vi "HEWH Close RLT Equipmet.vi"(7 "Semiphore":T1, 8 "Error In":errorcluster, 11 "RLT Equipment":T2={"COM A"="COM3", "MW100"="MW100", "AG34970"="A-34972A", "COM B"="COM4", "COM C"="COM5", "COM D"="COM6"}) -> (0 "Error Out":errorcluster)   [LabVIEW 2012]
uses:
  Drivers/Agilent 34970/Agilent 34970.lvlib
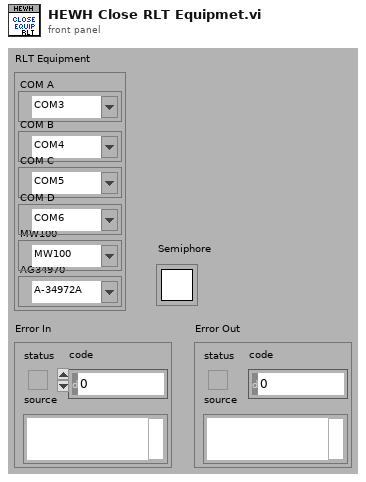
[diagram p1: front panel]
types:
  T1 = typedef "Semaphore RefNum" = refnum<k1>
  T2 = cluster{"COM A":refnum<visa-resource-name>, "MW100":refnum<visa-resource-name>, "AG34970":refnum<visa-resource-name>, "COM B":refnum<visa-resource-name>, "COM C":refnum<visa-resource-name>, "COM D":refnum<visa-resource-name>}
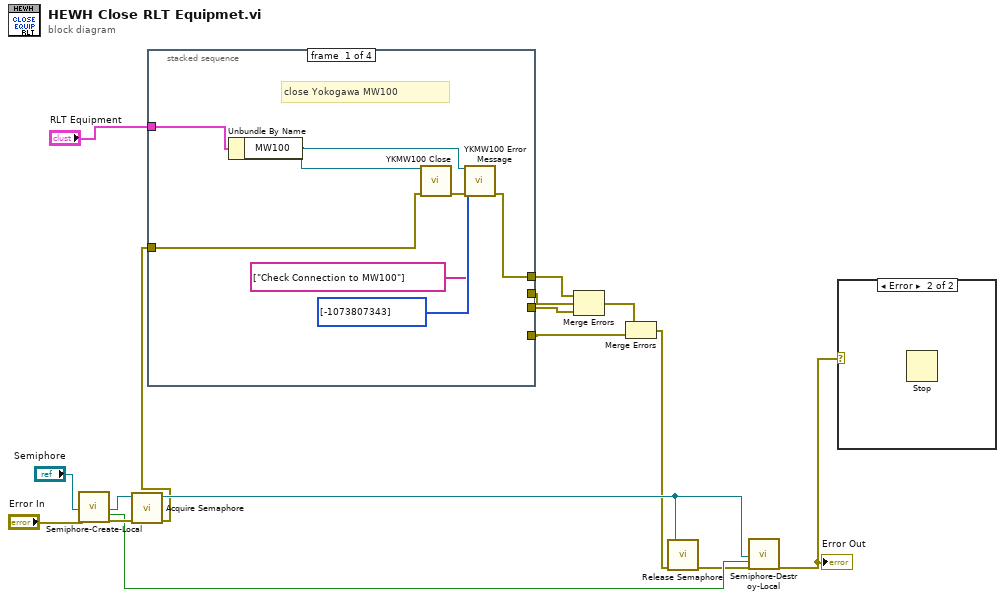
[diagram p0: block diagram]
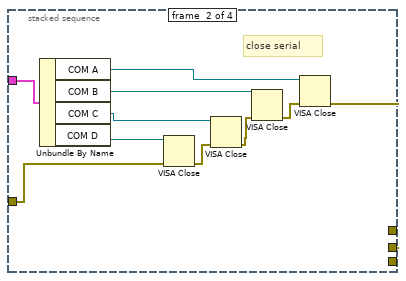
[diagram p3: hidden frame]
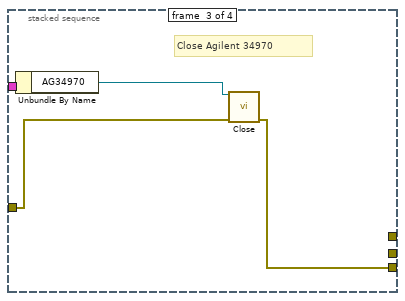
[diagram p4: hidden frame]
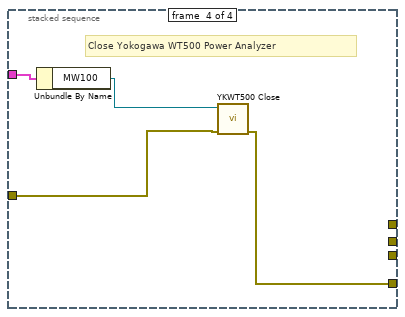
[diagram p5: hidden frame]
diagram:
  n1 = call "Semiphore-Create-Local.vi"("Semiphore"="Semiphore", "error in (no error)"="Error In") -> ("semaphore"=w9:T1, "Local?"=w6:bool, "error out"=w8:errorcluster)  [unwired: 15 in]
  n2 = call <vilib>:"Acquire Semaphore.vi"("error in (no error)"=w8, "semaphore"=w9) -> ("error out"=w3:errorcluster, "semaphore out"=w7:T1)  [unwired: 3 in, 1 out]
  n3 = stacked-sequence {
    tunnel: "RLT Equipment" -> [w23 w33 w37 w41]
    tunnel: [_ _ _ w40] -> w12
    tunnel: w3 -> [w22 w27 w35 w38]
    tunnel: [w20 _ _ _] -> w16
    tunnel: [_ w31 _ _] -> w15
    tunnel: [_ _ w34 _] -> w14
    frame #0 {
      # "close Yokogawa MW100"
      n4 = Unbundle By Name(w23) -> ("MW100"=w19:refnum<visa-resource-name>)
      n5 = call "YKMW100 Close.vi"("VISA session"=w19, "error in (no error)"=w22) -> ("error out"=w21:errorcluster)  [unwired: 13 in]
      n6 = call "YKMW100 Error Message.vi"("VISA session"=w19, "User-Defined Descriptions"=string[] ["Check Connection to MW100"], "User-Defined Codes"=i32[] [-1073807343], "error in (no error)"=w21) -> ("error out"=w20:errorcluster)  [unwired: 7 in, 4 out]
    }
    frame #1 {
      # "close serial"
      n7 = Unbundle By Name(w33) -> ("COM A"=w32:refnum<visa-resource-name>, "COM B"=w24:refnum<visa-resource-name>, "COM C"=w25:refnum<visa-resource-name>, "COM D"=w26:refnum<visa-resource-name>)
      n8 = VISA Close(VISA resource name=w26, error in (no error)=w27) -> (error out=w29:errorcluster)
      n9 = VISA Close(VISA resource name=w25, error in (no error)=w29) -> (error out=w28:errorcluster)
      n10 = VISA Close(VISA resource name=w24, error in (no error)=w28) -> (error out=w30:errorcluster)
      n11 = VISA Close(VISA resource name=w32, error in (no error)=w30) -> (error out=w31:errorcluster)
    }
    frame #2 {
      # "Close Agilent 34970"
      n12 = Unbundle By Name(w37) -> ("AG34970"=w36:refnum<visa-resource-name>)
      n13 = call "Close.vi"("VISA Resource Name"=w36, "error in (no error)"=w35) -> ("error out"=w34:errorcluster)  [unwired: 13 in]
    }
    frame #3 {
      # "Close Yokogawa WT500 Power Analyzer"
      n14 = Unbundle By Name(w41) -> ("MW100"=w39:refnum<visa-resource-name>)
      n15 = call "YKWT500 Close.vi"("error in (no error)"=w38, "VISA resource name"=w39) -> ("error out"=w40:errorcluster)  [unwired: 9 in]
    }
  }
  n16 = Merge Errors(w16, w15, w14) -> (w13:errorcluster)
  n17 = Merge Errors(w13, w12) -> (w2:errorcluster)
  n18 = call <vilib>:"Release Semaphore.vi"("error in (no error)"=w2, "semaphore"=w7) -> ("error out"=w5:errorcluster)  [unwired: 4 in, 1 out]
  n19 = call "Semiphore-Destroy-Local.vi"("Semiphore"=w7, "Local?"=w6, "error in (no error)"=w5) -> ("error out"=w1:errorcluster)  [unwired: 16 in]
  "Error Out" <- w1
  n20 = case shown="Error" w1 {
    frame No Error {
    }
    frame Error {
      n21 = Stop() -> ()  [unwired: 1 in]
    }
  }
